vi "AD7609 Get Nsamples.vi"() -> (1 "Channel volts":sgl[][](array[numeric]), 2 "error out":errorcluster)   [LabVIEW 2016]
uses:
  <vilib>/Instr/_visa.llb/VISA Open Access Mode.ctl
  AD7609 global.vi
panel:
  out "Channel data":cluster{sgl, sgl, sgl[][]}(graph)={0.0, 2.6666667e-05, []}
  # "PN 25/11/2014,  17/08/2015 (check for stop ack),\n23/08/2016 (timeout)"
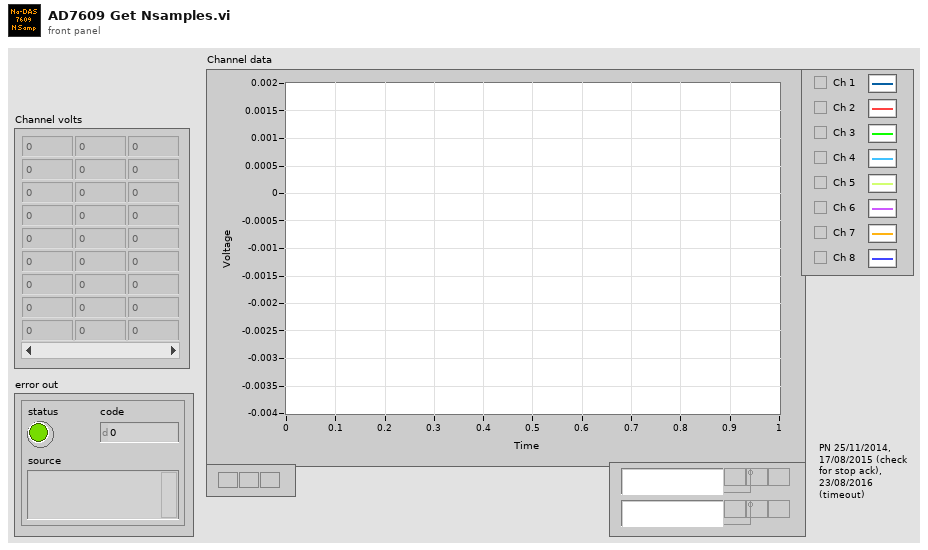
[diagram p1: front panel]
types:
  T1 = typedef "VISA Open Access Mode.ctl" = u32
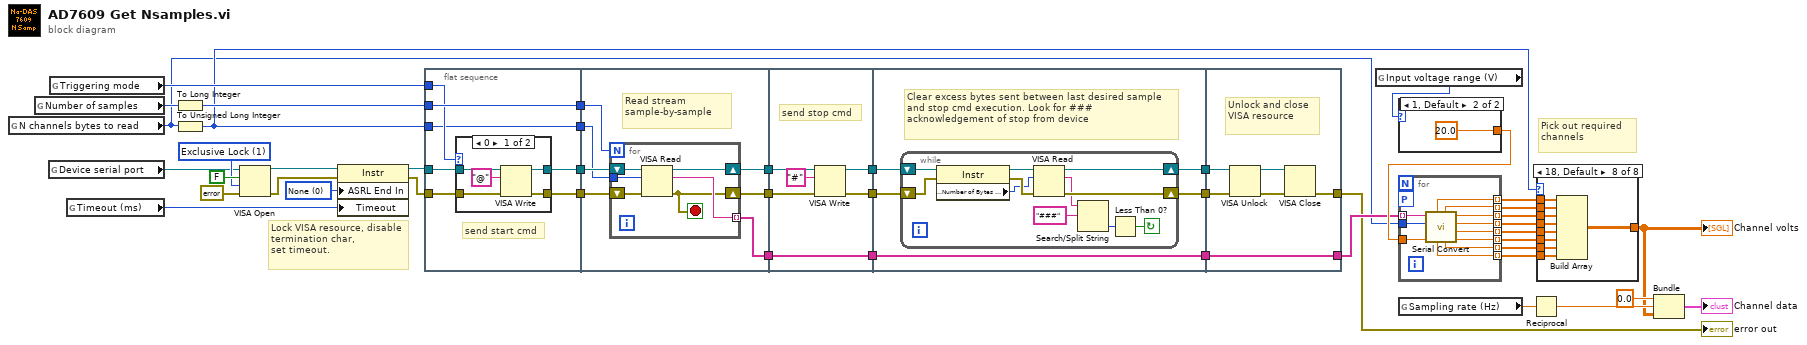
[diagram p0: block diagram]
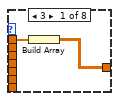
[diagram p2: hidden frame]
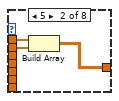
[diagram p3: hidden frame]
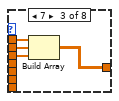
[diagram p4: hidden frame]
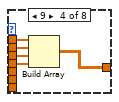
[diagram p5: hidden frame]
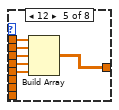
[diagram p6: hidden frame]
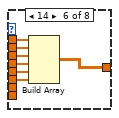
[diagram p7: hidden frame]
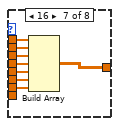
[diagram p8: hidden frame]
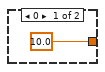
[diagram p9: hidden frame]
diagram:
  w2 = u16 0 items=["None", "Last Bit", "TermChar"] ("Serial Settings:End Mode for Reads")
  w43 = T1 1 items=["VISA Defaults"=0, "Exclusive Lock"=1, "Load Configured Settings"=4] ("Access Mode")
  # "Pick out required channels"
  # "Lock VISA resource, disable termination char,\nset timeout."
  n1 = global read "AD7609 global.vi" "N channels bytes to read"() -> (w8:u8)
  n2 = global read "AD7609 global.vi" "Number of samples"() -> (w21:u32)
  n3 = global read "AD7609 global.vi" "Device serial port"() -> (w7:refnum<visa-resource-name>)
  n4 = global read "AD7609 global.vi" "Triggering mode"() -> (w18:u8)
  n5 = global read "AD7609 global.vi" "Timeout (ms)"() -> (w1:u32)
  n6 = To Long Integer(number=w21) -> (32bit integer=w37:i32)
  n7 = To Unsigned Long Integer(number=w8) -> (unsigned 32bit integer=w16:u32)
  n8 = VISA Open(duplicate session (F)=FALSE, access mode=w43, error in (no error)=errorcluster {"status"=FALSE, "code"=0, "source"=""}, VISA resource name=w7) -> (VISA resource name=w6:refnum<visa-resource-name>, error out=w5:errorcluster)  [unwired: 1 in]
  n9 = property class="Instr"(reference=w6, error in=w5, "ASRL End In"=w2, "Timeout"=w1) -> (reference out=w4:refnum<visa-resource-name>, error out=w3:errorcluster)
  n10 = flat-sequence {
    tunnel: w3 -> [w52]
    tunnel: w4 -> [w51]
    tunnel: [w50] -> w42
    tunnel: [w49] -> w39
    tunnel: [w48] -> w38
    tunnel: w37 -> [w48]
    tunnel: w18 -> [w47]
    tunnel: w16 -> [w46]
    tunnel: [w46] -> w17
    tunnel: w42 -> [w66]
    tunnel: [w65] -> w41
    tunnel: [w64] -> w40
    tunnel: w39 -> [w63]
    tunnel: w38 -> [w62]
    tunnel: [w61] -> w36
    tunnel: w17 -> [w60]
    tunnel: w41 -> [w77]
    tunnel: w40 -> [w78]
    tunnel: [w74] -> w12
    tunnel: w36 -> [w74]
    tunnel: [w76] -> w13
    tunnel: [w75] -> w14
    tunnel: w14 -> [w79]
    tunnel: w13 -> [w82]
    tunnel: w12 -> [w83]
    tunnel: [w83] -> w11
    tunnel: [w81] -> w10
    tunnel: [w80] -> w9
    tunnel: w11 -> [w97]
    tunnel: [w98] -> w19
    tunnel: [w97] -> w20
    tunnel: w10 -> [w96]
    tunnel: w9 -> [w95]
    frame #0 {
      # "send start cmd"
      n11 = case shown="0" w47 {
        tunnel: w52 -> [w56 w58]
        tunnel: w51 -> [w55 w59]
        tunnel: [w54 w58] -> w50
        tunnel: [w53 w59] -> w49
        frame 0 {
          n12 = VISA Write(VISA resource name=w55, write buffer="@", error in (no error)=w56) -> (VISA resource name out=w53:refnum<visa-resource-name>, error out=w54:errorcluster)  [unwired: 1 out]
        }
        frame Default {
        }
      }
    }
    frame #1 {
      # "Read stream sample-by-sample"
      n13 = for {
        N: w62 -> [_]
        shift-right: [w67] -> w65
        shift-left: w66 -> [w72]
        shift-right: [w71] -> w64
        shift-left: w63 -> [w70]
        tunnel: [w69] -> w61 mode=indexing
        tunnel: w60 -> [w68]
        stop <- w67 stop-if-true
        n14 = VISA Read(VISA resource name=w70, byte count=w68, error in (no error)=w72) -> (VISA resource name out=w71:refnum<visa-resource-name>, read buffer=w69:string, error out=w67:errorcluster)  [unwired: 1 out]
      }
    }
    frame #2 {
      # "send stop cmd"
      n15 = VISA Write(VISA resource name=w78, write buffer="#", error in (no error)=w77) -> (VISA resource name out=w76:refnum<visa-resource-name>, error out=w75:errorcluster)  [unwired: 1 out]
    }
    frame #3 {
      # "Clear excess bytes sent between last desired sample  and stop cmd execution. Look for ### acknowledgement of stop from device"
      n16 = while {
        shift-right: [w90] -> w81
        shift-left: w79 -> [w93]
        shift-right: [w89] -> w80
        shift-left: w82 -> [w94]
        stop <- w85 continue-if-true
        n17 = property class="Instr"(reference=w94, error in=w93) -> (reference out=w92:refnum<visa-resource-name>, error out=w91:errorcluster, "Serial Settings:Number of Bytes at Serial Port"=w84:u32)
        n18 = VISA Read(VISA resource name=w92, byte count=w84, error in (no error)=w91) -> (VISA resource name out=w89:refnum<visa-resource-name>, read buffer=w88:string, error out=w90:errorcluster)  [unwired: 1 out]
        n19 = Search/Split String(string=w88, search string/char (-)="###") -> (offset of match=w86:i32)  [unwired: 1 in, 2 out]
        n20 = Less Than 0?(x=w86) -> (x < 0?=w85:bool)
      }
    }
    frame #4 {
      # "Unlock and close VISA resource"
      n21 = VISA Unlock(8:w96, 11:w95) -> (0:w100:errorcluster, 3:w99:refnum<visa-resource-name>)
      n22 = VISA Close(VISA resource name=w99, error in (no error)=w100) -> (error out=w98:errorcluster)
    }
  }
  n23 = global read "AD7609 global.vi" "Input voltage range (V)"() -> (w31:u8)
  n24 = case shown="1, Default" w31 {
    tunnel: [sgl 10.0 sgl 20.0] -> w32
    frame 0 {
    }
    frame 1, Default {
    }
  }
  n25 = for {
    tunnel: w20 -> [w113] mode=indexing
    tunnel: w32 -> [w112]
    tunnel: [w111] -> w30 mode=indexing
    tunnel: [w110] -> w29 mode=indexing
    tunnel: [w109] -> w28 mode=indexing
    tunnel: [w108] -> w27 mode=indexing
    tunnel: [w107] -> w26 mode=indexing
    tunnel: [w106] -> w25 mode=indexing
    tunnel: [w105] -> w24 mode=indexing
    tunnel: [w104] -> w23 mode=indexing
    workers-P: _ -> [_]
    tunnel: w8 -> [w103]
    n26 = call "Serial Convert.vi"("Range (V)"=w112, "N channels bytes to read"=w103, "Raw serial buffer"=w113) -> ("V6 (V)"=w106:sgl, "V5 (V)"=w107:sgl, "V4 (V)"=w108:sgl, "V3 (V)"=w109:sgl, "V7 (V)"=w105:sgl, "V2 (V)"=w110:sgl, "V8 (V)"=w104:sgl, "V1 (V)"=w111:sgl)  [unwired: 1 in]
  }
  n27 = global read "AD7609 global.vi" "Sampling rate (Hz)"() -> (w34:sgl)
  n28 = Reciprocal(x=w34) -> (1/x=w33:sgl)
  n29 = case shown="18, Default" w16 {
    tunnel: w30 -> [w115 w118 w122 w127 w133 w140 w148 w157]
    tunnel: w29 -> [_ w116 w121 w126 w132 w139 w147 w156]
    tunnel: w28 -> [_ _ w120 w125 w131 w138 w146 w155]
    tunnel: w27 -> [_ _ _ w124 w130 w137 w145 w154]
    tunnel: w26 -> [_ _ _ _ w129 w136 w144 w153]
    tunnel: w25 -> [_ _ _ _ _ w135 w143 w152]
    tunnel: w24 -> [_ _ _ _ _ _ w142 w151]
    tunnel: w23 -> [_ _ _ _ _ _ _ w150]
    tunnel: [w114 w117 w119 w123 w128 w134 w141 w149] -> w22
    frame 3 {
      n30 = Build Array(w115) -> (w114:sgl[][])
    }
    frame 5 {
      n31 = Build Array(w118, w116) -> (w117:sgl[][])
    }
    frame 7 {
      n32 = Build Array(w122, w121, w120) -> (w119:sgl[][])
    }
    frame 9 {
      n33 = Build Array(w127, w126, w125, w124) -> (w123:sgl[][])
    }
    frame 12 {
      n34 = Build Array(w133, w132, w131, w130, w129) -> (w128:sgl[][])
    }
    frame 14 {
      n35 = Build Array(w140, w139, w138, w137, w136, w135) -> (w134:sgl[][])
    }
    frame 16 {
      n36 = Build Array(w148, w147, w146, w145, w144, w143, w142) -> (w141:sgl[][])
    }
    frame 18, Default {
      n37 = Build Array(w157, w156, w155, w154, w153, w152, w151, w150) -> (w149:sgl[][])
    }
  }
  "Channel volts" <- w22
  n38 = Bundle(sgl 0.0, w33, w22) -> (→"Channel data":cluster{sgl, sgl, sgl[][]})  [unwired: 1 in]
  "error out" <- w19
